vi "test zernike.vi"() -> ()   [LabVIEW 2012]
uses:
  LightPipes.lvlib
panel:
  in  "A":dbl=10.0
  in  "R":dbl=0.01
  in  "m":i32=1
  in  "n":i32=3
  out "Wave Front":dbl[][](graph)
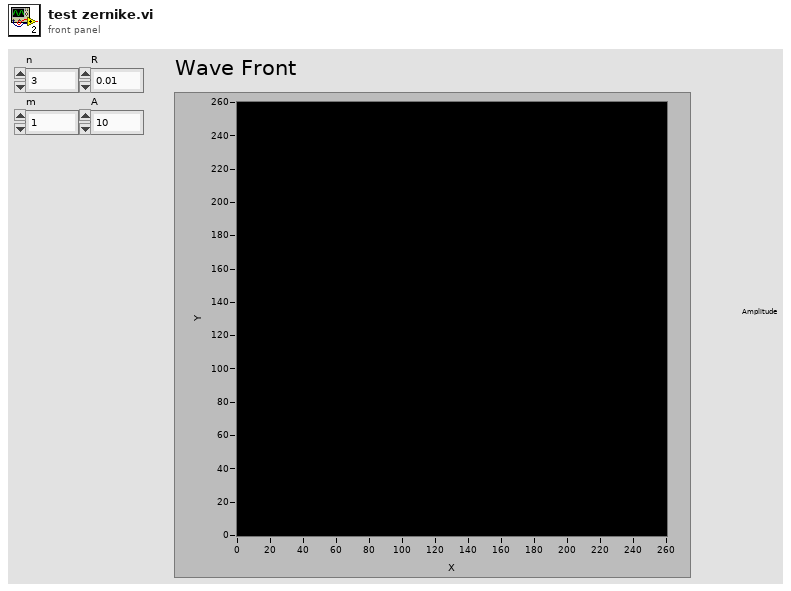
[diagram p1: front panel]
types:
  T1 = cluster{"n_grid":i32, "@dummy control@":i8, "@dummy control@":i8, "@dummy control@":i8, "@dummy control@":i8, "size":dbl, "lambda":dbl, "int1":i32, "int2":i32, "int3":i32, "@dummy control@":i8, "@dummy control@":i8, "@dummy control@":i8, "@dummy control@":i8, "double1":dbl, "double2":dbl, "double3":dbl, "real":u32, "imaginary":u32}
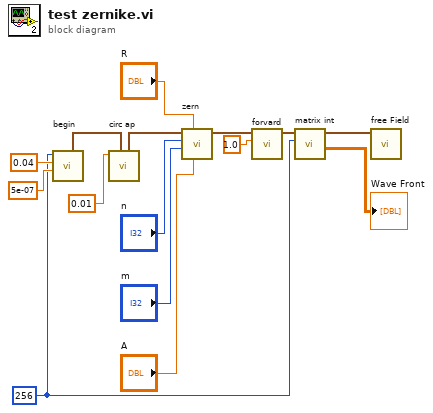
[diagram p0: block diagram]
diagram:
  w9 = 256 ("n_grid")
  n1 = call "begin.vi"("lambda"=5e-07, "size_grid"=0.04, "n_grid"=w9) -> ("field out"=w13:T1)  [unwired: 8 in]
  n2 = call "circ ap.vi"("field"=w13, "radius"=0.01) -> ("field out"=w12:T1)  [unwired: 9 in]
  n3 = call "zern.vi"("A"="A", "R"="R", "m"="m", "n"="n", "field"=w12) -> ("field out"=w3:T1)  [unwired: 6 in]
  n4 = call "forvard.vi"("distance"=1.0, "field"=w3) -> ("field out"=w2:T1)  [unwired: 9 in]
  n5 = call "matrix int.vi"("n_grid"=w9, "field"=w2) -> ("matrix out 2D"=→"Wave Front":dbl[][], "field out"=w10:T1)  [unwired: 8 in]
  n6 = call "free Field.vi"("field"=w10) -> ()  [unwired: 10 in, 1 out]
